vi "Shutdown.vi"(8 "error in (no error)":errorcluster, 11 "Thermocouple in":refnum<class "Thermocouple.lvclass">) -> (0 "error out":errorcluster, 3 "Thermocouple out":refnum<class "Thermocouple.lvclass">)   [LabVIEW 2018, in "Thermocouple.lvlib" / "Thermocouple.lvclass"]
uses:
  Thermocouple.lvclass
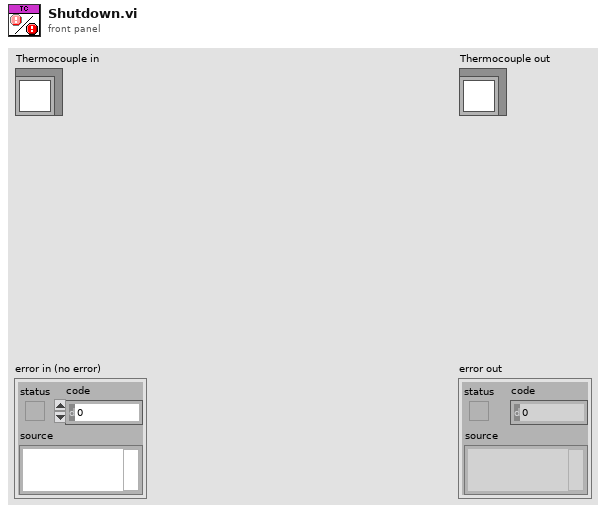
[diagram p1: front panel]
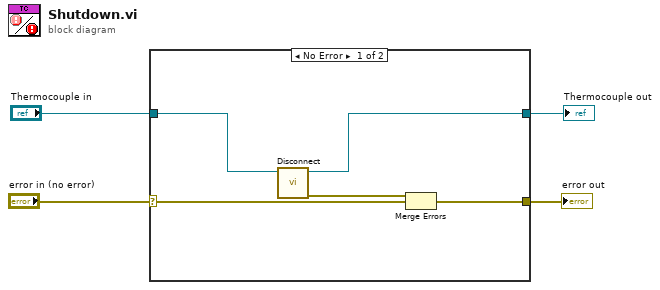
[diagram p0: block diagram]
diagram:
  n1 = case shown="No Error" "error in (no error)" {
    selector: "error in (no error)" -> [w6 w11]
    tunnel: [w5 w11] -> w3
    tunnel: [w7 w10] -> w1
    tunnel: "Thermocouple in" -> [w8 w10]
    frame No Error {
      n2 = call-dynamic "Disconnect.vi"("Thermocouple in"=w8) -> ("error out"=w9:errorcluster, "Thermocouple out"=w7:refnum<class "Thermocouple.lvclass">)  [unwired: 9 in]
      n3 = Merge Errors(w9, w6) -> (w5:errorcluster)
    }
    frame Error {
    }
  }
  "error out" <- w3
  "Thermocouple out" <- w1
